vi "macro_PIDController_AdvExecute.vi"   [LabVIEW 2019, in "Trajectory_Library.lvlib"]
uses:
  Trajectory_Library.lvlib
types:
  T1 = typedef "Trajectory_Library.lvlib/PID_ADV_LIMITS.ctl" = cluster{"MaxInput":dbl, "MinInput":dbl, "Continuous":bool, "MaxOutput":dbl, "MinOutput":dbl}
  T2 = typedef "Trajectory_Library.lvlib/PID_ADV_TUNING.ctl" = cluster{"Kf":dbl, "Kp":dbl, "Ki":dbl, "Kd":dbl, "MaximumIntegral":dbl, "MinimumIntegral":dbl, "Filter Derivative":bool}
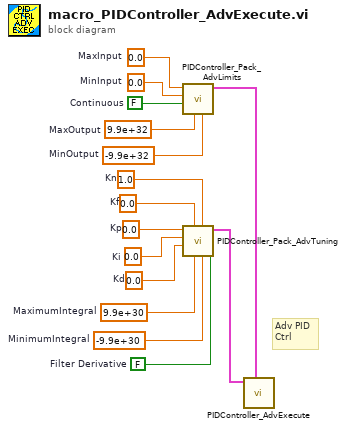
[diagram p0: block diagram]
diagram:
  w1 = 1.0  # Kn
  w2 = 0.0  # Kp
  w3 = 0.0  # Ki
  w4 = 0.0  # Kd
  w5 = 0.0  # Kf
  w6 = 9.9e+30  # MaximumIntegral
  w7 = -9.9e+30  # MinimumIntegral
  w8 = FALSE  # Filter Derivative
  w10 = 0.0  # MinInput
  w11 = FALSE  # Continuous
  w12 = 9.9e+32  # MaxOutput
  w9 = -9.9e+32  # MinOutput
  w13 = 0.0  # MaxInput
  # "Adv PID\nCtrl"
  n1 = call "PIDController_Pack_AdvLimits.vi"("MinOutput"=w9, "MaxOutput"=w12, "Continuous"=w11, "MinInput"=w10, "MaxInput"=w13) -> ("Adv PID Limits"=w15:T1)  [unwired: 6 in]
  n2 = call "PIDController_Pack_AdvTuning.vi"("Filter Derivative"=w8, "MinimumIntegral"=w7, "Kn"=w1, "MaximumIntegral"=w6, "Kf"=w5, "Kd"=w4, "Ki"=w3, "Kp"=w2) -> ("Adv PID Tuning"=w14:T2)  [unwired: 3 in]
  n3 = call "PIDController_AdvExecute.vi"("Adv PID Limits"=w15, "Adv PID Tuning"=w14) -> ()  [unwired: 7 in, 3 out]
